vi "opCRD Server (9636).vi"   [LabVIEW 2015]
uses:
  Reusable/Session Log/System Log.lvclass
  Reusable/Session Log/System Log.lvclass/System Log.ctl
  <vilib>/Platform/TimedLoop/XDataNode/timing_clust.ctl
  <vilib>/Platform/TimedLoop/XDataNode/nitl_modes.ctl
  <vilib>/Platform/TimedLoop/XDataNode/wakeup.ctl
  Reusable/Session Log/Accessors/Write Main Path.vi
  <vilib>/nisyscfg/Close (System).vi
  <userlib>/_Session Fwk/Session - Root.lvclass
  <vilib>/Platform/TimedLoop/XDataNode/XDataNode.xnode
  <vilib>/Platform/TimedLoop/XDataNode/XDNodeRunTimeDep.lvlib
  <vilib>/nisyscfg/nisyscfg.lvlib
types:
  T1 = typedef "XDNodeRunTimeDep.lvlib/timing_clust.ctl" = cluster{"Expected End [f-1]":u64, "Actual End [f-1]":u64, "Finished Late? [f-1]":bool, "Expected End [i-1]":u64, "Actual End [i-1]":u64, "Finished Late? [i-1]":bool, "Expected Start [i]":u64, "Actual Start [i]":u64, "Expected Start [f]":u64, "Actual Start [f]":u64, "Source Name":string, "Structure Name":string, "Period":i64, "Deadline":i64, "Offset":i64, "Start":i64, "Priority":i32, "Timeout":i32, "Mode":T2, "Wakeup Reason":T3, "Error":errorcluster, "Source Type":string, "Secondary Source Type":string, "Global End Time":u64, "Global Start Time":u64, "Frame Duration":u64, "Iteration Duration":u64, "Assigned CPU":i32, "I/O Scan Engine Mode":u32}
  T2 = typedef "XDNodeRunTimeDep.lvlib/nitl_modes.ctl" = enum32{"No Change", "Process missed periods, maintain original phase", "Discard missed periods, maintain original phase", "Process missed periods, ignore original phase", "Discard missed periods, ignore original phase"}
  T3 = typedef "XDNodeRunTimeDep.lvlib/wakeup.ctl" = enum32{"Normal", "Aborted", "Asynchronous wakeup", "Timing source error", "Timed loop error", "Timeout"}
  T4 = typedef "Session - Root.lvclass/Session Handle.ctl" = refnum<data-value>
  T5 = typedef "LVDateTimeRec.ctl" = cluster{"fractional second":dbl, "second":i32, "minute":i32, "hour":i32, "day of month":i32, "month":i32, "year":i32, "day of week":i32, "day of year":i32, "DST":i32}
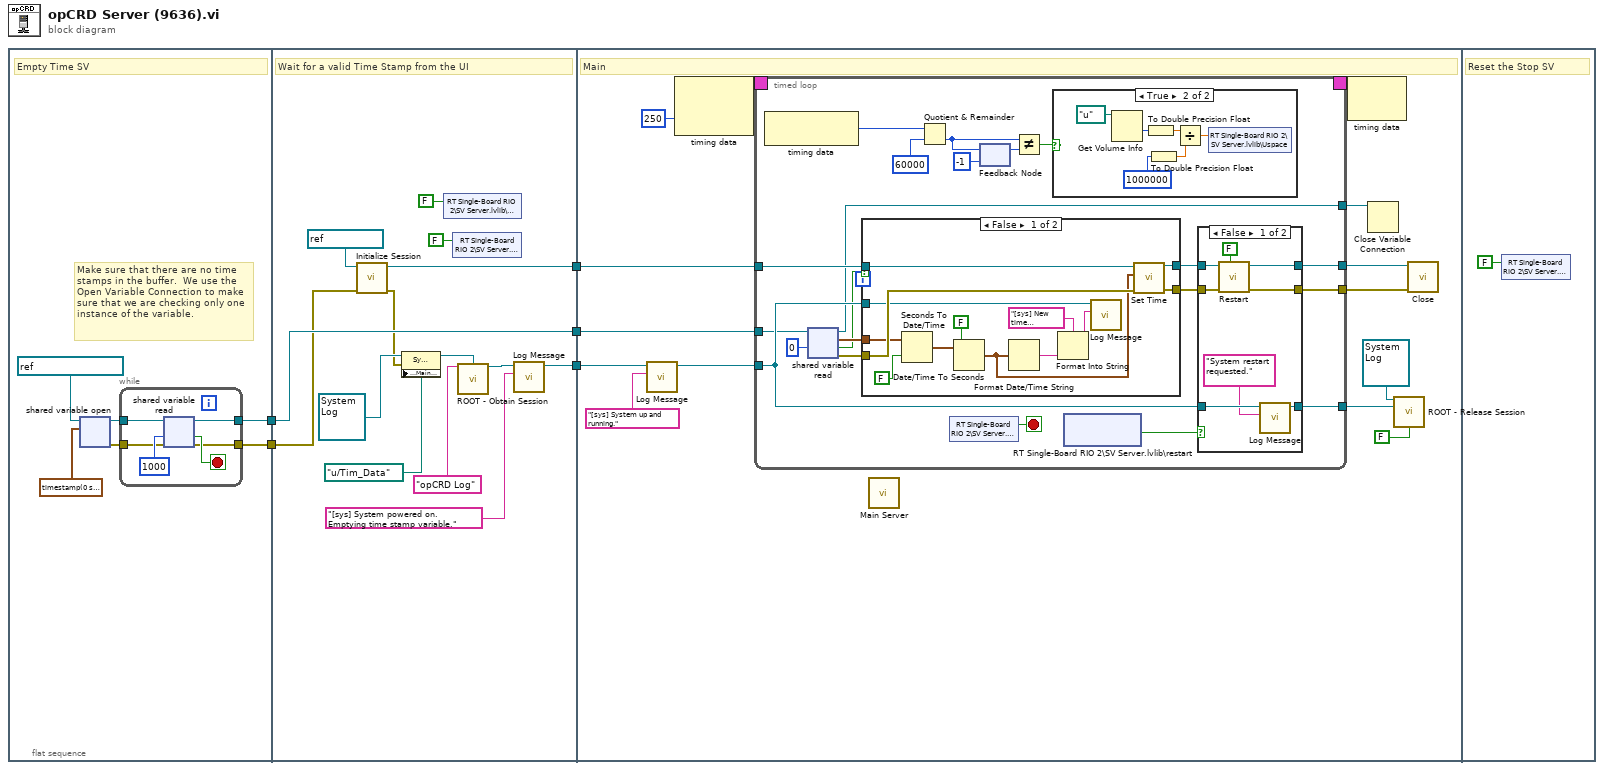
[diagram p0: block diagram]
diagram:
  n1 = flat-sequence {
    tunnel: [w11] -> w5
    tunnel: [w10] -> w4
    tunnel: [w31] -> w3
    tunnel: w5 -> [w24]
    tunnel: w4 -> [w23]
    tunnel: [w20] -> w2
    tunnel: [w24] -> w1
    tunnel: w3 -> [w40]
    tunnel: w2 -> [w39]
    tunnel: w1 -> [w37]
    frame #0 {
      # "Make sure that there are no time stamps in the buffer.  We use the Open Variable Connection to make sure that we are checking only one instance of the variable."
      # "Empty Time SV"
      n2 = shared-variable-open(refnum<k21> "ni.var.psp://rt single-board rio 2/SV Server/Time" ("shared variable refnum in"), timestamp(0 s since 1904-01-01)) -> (w8:refnum<k21>, w6:errorcluster)  [unwired: 2 in]
      n3 = while {
        tunnel: [w13] -> w10
        tunnel: w8 -> [w17]
        tunnel: [w14] -> w11
        tunnel: w6 -> [w12]
        stop <- w15 stop-if-true
        n4 = shared-variable-read(w17, w12, 1000 ("timeout ms")) -> (w14:refnum<k21>, w13:errorcluster, w15:bool)  [unwired: 2 out]
      }
    }
    frame #1 {
      # "Wait for a valid Time Stamp from the UI"
      n5 = call <vilib>:"Initialize Session.vi"("error in (no error)"=w23, "Target (localhost)"=refnum<k21> "localhost" ("target (localhost)")) -> ("error out"=w21:errorcluster, "Session out"=w31:refnum<k21>)  [unwired: 8 in]
      n6 = property class="Sys Log"(reference=refnum<class "System Log.lvclass"> refnum ("Sys Log"), error in=w21, "Accessors:Main Path"=path "u:/Tim_Data" ("RD Data Path")) -> (reference out=w26:refnum<class "System Log.lvclass">)  [unwired: 1 out]
      n7 = shared-variable "RT Single-Board RIO 2\\SV Server.lvlib\\Write?"(FALSE ("Write?")) -> ()  [unwired: 1 in, 1 out]
      n8 = shared-variable "RT Single-Board RIO 2\\SV Server.lvlib\\Stop"(FALSE ("Stop")) -> ()  [unwired: 1 in, 1 out]
      n9 = call <userlib>:"ROOT - Obtain Session.vi"("Session Name ()"="opCRD Log", "OBJ - Session"=w26) -> ("Session Handle"=w28:T4)  [unwired: 11 in, 2 out]
      n10 = call "Log Message.vi"("MSG In"="[sys] System powered on.  Emptying time stamp variable.", "session in"=w28) -> ("session out"=w20:T4)  [unwired: 8 in, 1 out]
    }
    frame #2 {
      # "Main"
      n11 = call "Log Message.vi"("MSG In"="[sys] System up and running.", "session in"=w39) -> ("session out"=w36:T4)  [unwired: 8 in, 1 out]
      n12 = node-c288(i64 250 ("Period")) -> (w45:T1)  [unwired: 1 in]
      n13 = timed-loop {
        timing: w45 -> [_]
        timing-out: [_] -> w44
        tunnel: w40 -> [w65]
        tunnel: [w63] -> w42
        tunnel: [w61] -> w41
        tunnel: w36 -> [w59]
        tunnel: w37 -> [w58]
        tunnel: [w53] -> w35
        tunnel: [w52] -> w32
        stop <- w66 stop-if-true
        n14 = node-c288() -> (w51:i64)  [unwired: 1 in]
        n15 = shared-variable-read(w58, 0 ("timeout ms")) -> (w53:refnum<k21>, w56:errorcluster, w54:bool, w55:timestamp)  [unwired: 1 in, 1 out]
        n16 = case shown="False" w54 {
          tunnel: w55 -> [w87 _]
          tunnel: w65 -> [w98 w100]
          tunnel: [w97 w100] -> w64
          tunnel: w56 -> [w96 w99]
          tunnel: [w95 w99] -> w62
          tunnel: w59 -> [w94 _]
          frame False {
            n17 = Seconds To Date/Time(time stamp (now)=w87, to UTC (F)=FALSE) -> (date time rec=w90:T5)
            n18 = Date/Time To Seconds(1:FALSE ("is UTC (F)"), 2:w90) -> (0:w86:timestamp)
            n19 = Format Date/Time String(seconds (now)=w86) -> (date/time string=w92:string)  [unwired: 2 in]
            n20 = Format Into String(format string="[sys] New time requested.  New time is %s." ("MSG In"), w92) -> (resulting string=w91:string)  [unwired: 2 in, 1 out]
            n21 = call "Log Message.vi"("MSG In"=w91, "session in"=w94) -> ()  [unwired: 8 in, 2 out]
            n22 = call <vilib>:"Set Time.vi"("error in (no error)"=w96, "Time"=w86, "Session in (localhost)"=w98) -> ("error out"=w95:errorcluster, "Session out"=w97:refnum<k21>)  [unwired: 5 in, 2 out]
          }
          frame True {
          }
        }
        n23 = Quotient & Remainder(x=w51, y=i64 60000) -> (floor(x/y)=w48:i64)  [unwired: 1 out]
        n24 = shared-variable "RT Single-Board RIO 2\\SV Server.lvlib\\Stop"() -> (w66:bool)  [unwired: 1 in, 1 out]
        n25 = feedback-in #1(w48) -> ()
        n26 = feedback #1(i64 -1) -> (w47:i64)
        n27 = Not Equal?(x=w48, y=w47) -> (x != y?=w46:bool)
        n28 = case shown="True" w46 {
          frame False {
          }
          frame True {
            n29 = Get Volume Info(11:path "u:/" ("path")) -> (1:w70:i64)  [unwired: 1 in, 5 out]
            n30 = To Double Precision Float(number=w70) -> (double precision float=w69:dbl)
            n31 = To Double Precision Float(number=i64 1000000 ("y")) -> (double precision float=w68:dbl)
            n32 = Divide(x=w69, y=w68) -> (x/y=w71:dbl)
            n33 = shared-variable "RT Single-Board RIO 2\\SV Server.lvlib\\Uspace"(w71) -> ()  [unwired: 1 in, 1 out]
          }
        }
        n34 = shared-variable "RT Single-Board RIO 2\\SV Server.lvlib\\restart"() -> (w60:bool)  [unwired: 2 in, 2 out]
        n35 = case shown="False" w60 {
          tunnel: w64 -> [w82 w85]
          tunnel: [w81 w85] -> w63
          tunnel: w62 -> [w79 w84]
          tunnel: [w78 w84] -> w61
          tunnel: w59 -> [w77 w83]
          tunnel: [w75 w83] -> w52
          frame False {
            n36 = call <vilib>:"Restart.vi"("Wait Until Complete (T)"=FALSE ("wait until complete (T)"), "error in (no error)"=w79, "Session in"=w82) -> ("error out"=w78:errorcluster, "Session out"=w81:refnum<k21>)  [unwired: 6 in, 1 out]
            n37 = call "Log Message.vi"("MSG In"="System restart requested.", "session in"=w77) -> ("session out"=w75:T4)  [unwired: 8 in, 1 out]
          }
          frame True {
          }
        }
      }
      n38 = call "Main Server.vi"() -> ()  [unwired: 11 in, 1 out]
      n39 = node-c288(w44) -> ()  [unwired: 1 out]
      n40 = Close Variable Connection(11:w35) -> ()  [unwired: 1 in, 1 out]
      n41 = call <userlib>:"ROOT - Release Session.vi"("OBJ - Session in"=refnum<class "System Log.lvclass"> refnum ("Sys Log"), "Session Handle in"=w32, "force destroy? (F)"=FALSE) -> ()  [unwired: 11 in, 2 out]
      n42 = call-poly <vilib>:"Close.vi"("error in (no error)"=w41, "Session in"=w42) -> ()  [unwired: 9 in, 1 out]
    }
    frame #3 {
      # "Reset the Stop SV"
      n43 = shared-variable "RT Single-Board RIO 2\\SV Server.lvlib\\Stop"(FALSE ("Stop")) -> ()  [unwired: 1 in, 1 out]
    }
  }
